vi "Format Cell Address.vi"(11 "Cell Address":string) -> (3 "Formatted Cell Address":string)   [LabVIEW 2019, in "Open Xml.lvlib"]
uses:
  Open Xml.lvlib
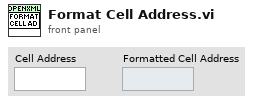
[diagram p1: front panel]
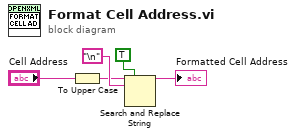
[diagram p0: block diagram]
diagram:
  n1 = To Upper Case(1:"Cell Address") -> (0:w2:string)
  n2 = Search and Replace String(replace all?=TRUE ("replace all? (F)"), input string=w2, search string="\n") -> (result string=→"Formatted Cell Address":string)  [unwired: 5 in, 3 out]
